vi "SIM Simulation Global Settings.vi"() -> ()   [LabVIEW 2012]
panel:
  out "Allow reverse time simulation?":bool
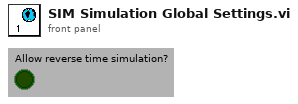
[diagram p1: front panel]
diagram:
